vi "Send.vi"(0 "Nom de ressource VISA":refnum<visa-resource-name>, 1 "Data":u8[](array[numeric]), 2 "Type":u8, 3 "entrée d'erreur (pas d'erreur)":errorcluster, 4 "Long_Data":i32) -> (5 "taille(s)":i32, 6 "sortie d'erreur":errorcluster)   [LabVIEW 2010]
doc: "Fonction d'envoi des données"
uses:
  <vilib>/Instr/_visa.llb/VISA Flush IO Buffer Mask.ctl
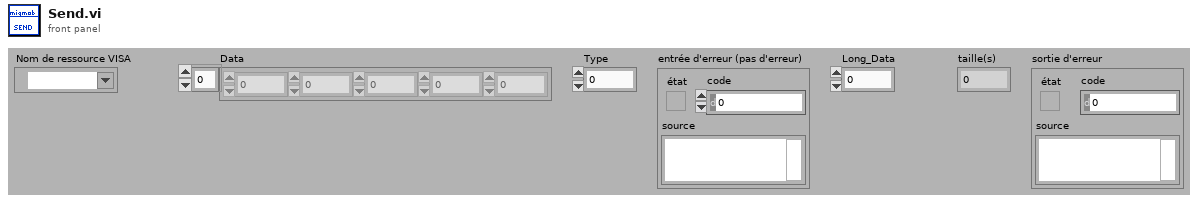
[diagram p1: front panel]
types:
  T1 = typedef "VISA Flush IO Buffer Mask.ctl" = u16
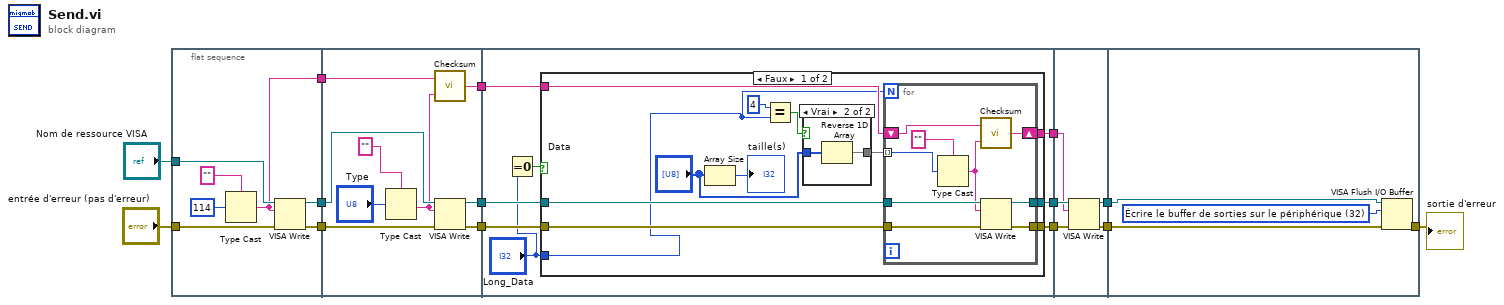
[diagram p0: block diagram]
diagram:
  n1 = flat-sequence {
    tunnel: "Nom de ressource VISA" -> [w21]
    tunnel: "entrée d'erreur (pas d'erreur)" -> [w20]
    tunnel: [w19] -> w14
    tunnel: [w18] -> w13
    tunnel: [w15] -> w12
    tunnel: w14 -> [w30]
    tunnel: w13 -> [w29]
    tunnel: [w26] -> w11
    tunnel: [w25] -> w10
    tunnel: w12 -> [w24]
    tunnel: [w22] -> w9
    tunnel: w11 -> [w35]
    tunnel: w10 -> [w36]
    tunnel: [w34] -> w8
    tunnel: [w33] -> w7
    tunnel: w9 -> [w38]
    tunnel: [w37] -> w6
    tunnel: w8 -> [w70]
    tunnel: w7 -> [w69]
    tunnel: w6 -> [w67]
    tunnel: [w68] -> w5
    tunnel: [w66] -> w4
    tunnel: [w71] -> w1
    tunnel: w5 -> [w72]
    tunnel: w4 -> [w73]
    frame #0 {
      n2 = Type Cast(type="", x=u8 114) -> (*(type *) &x=w15:string)
      n3 = VISA Write(VISA resource name=w21, write buffer=w15, error in (no error)=w20) -> (VISA resource name out=w19:refnum<visa-resource-name>, error out=w18:errorcluster)  [unwired: 1 out]
    }
    frame #1 {
      n4 = Type Cast(type="", x="Type") -> (*(type *) &x=w23:string)
      n5 = call "Checksum.vi"("Byte2"=w23, "Byte1"=w24) -> ("chaîne"=w22:string)
      n6 = VISA Write(VISA resource name=w30, write buffer=w23, error in (no error)=w29) -> (VISA resource name out=w25:refnum<visa-resource-name>, error out=w26:errorcluster)  [unwired: 1 out]
    }
    frame #2 {
      n7 = Equal To 0?(x="Long_Data") -> (x = 0?=w32:bool)
      n8 = case shown="Faux" w32 {
        tunnel: w38 -> [w50 w65]
        tunnel: [w49 w65] -> w37
        tunnel: w36 -> [w44 w64]
        tunnel: w35 -> [w43 w63]
        tunnel: [w42 w64] -> w34
        tunnel: [w41 w63] -> w33
        tunnel: "Long_Data" -> [w39 _]
        frame False {
          n9 = Array Size(array="Data") -> (size(s)=→"taille(s)":i32)
          n10 = Equal?(x=4, y=w39) -> (x = y?=w47:bool)
          n11 = case shown="Vrai" w47 {
            tunnel: "Data" -> [w51 w53]
            tunnel: [w51 w52] -> w45
            frame False {
            }
            frame True {
              n12 = Reverse 1D Array(array=w53) -> (reversed array=w52:u8[])
            }
          }
          n13 = for {
            N: w39 -> [_]
            shift-right: [w61] -> w49
            shift-left: w50 -> [w62]
            tunnel: w45 -> [w59] mode=indexing
            tunnel: w44 -> [w58]
            tunnel: w43 -> [w57]
            tunnel: [w55] -> w42
            tunnel: [w54] -> w41
            n14 = Type Cast(type="", x=w59) -> (*(type *) &x=w56:string)
            n15 = call "Checksum.vi"("Byte2"=w56, "Byte1"=w62) -> ("chaîne"=w61:string)
            n16 = VISA Write(VISA resource name=w58, write buffer=w56, error in (no error)=w57) -> (VISA resource name out=w55:refnum<visa-resource-name>, error out=w54:errorcluster)  [unwired: 1 out]
          }
        }
        frame True {
        }
      }
    }
    frame #3 {
      n17 = VISA Write(VISA resource name=w70, write buffer=w67, error in (no error)=w69) -> (VISA resource name out=w66:refnum<visa-resource-name>, error out=w68:errorcluster)  [unwired: 1 out]
    }
    frame #4 {
      w74 = T1 32 items=["Vider le buffer d'entrées"=16, "Écrire le buffer de sorties sur le périphérique"=32, "Vider le buffer d'entrées (Pas d'E/S)"=64, "Vider le buffer de sorties"=128] ("Mask")
      n18 = VISA Flush I/O Buffer(VISA resource name=w73, mask (16)=w74, error in (no error)=w72) -> (error out=w71:errorcluster)  [unwired: 1 out]
    }
  }
  "sortie d'erreur" <- w1
